vi "S2DS_EditFormula.vi"(8 "error in (no error)":errorcluster, 10 "WC info out":T2, 11 "formula in":string) -> (0 "error out":errorcluster, 1 "Parsed Formula Node (out)":T1, 3 "formula (out)":string)   [LabVIEW 2025]
uses:
  TYPE DEFS/S2DS_WC info.ctl
  TYPE DEFS/S2DS_Single WC info.ctl
  <vilib>/gmath/NI_Gmath.lvlib
panel:
  in  "Original formula":bool
  in  "Clear error":bool
  in  "OK":bool
  out "error":errorcluster
  in  "Quit sweep":bool
  out "Channel assignment":string[][](array[string])
  out "Output":dbl[](array[numeric]) format="%.2f"
  in  "Input":dbl[](array[numeric]) format="%.2f"
  in  "formula":string
  # "EDIT FORMULA..."
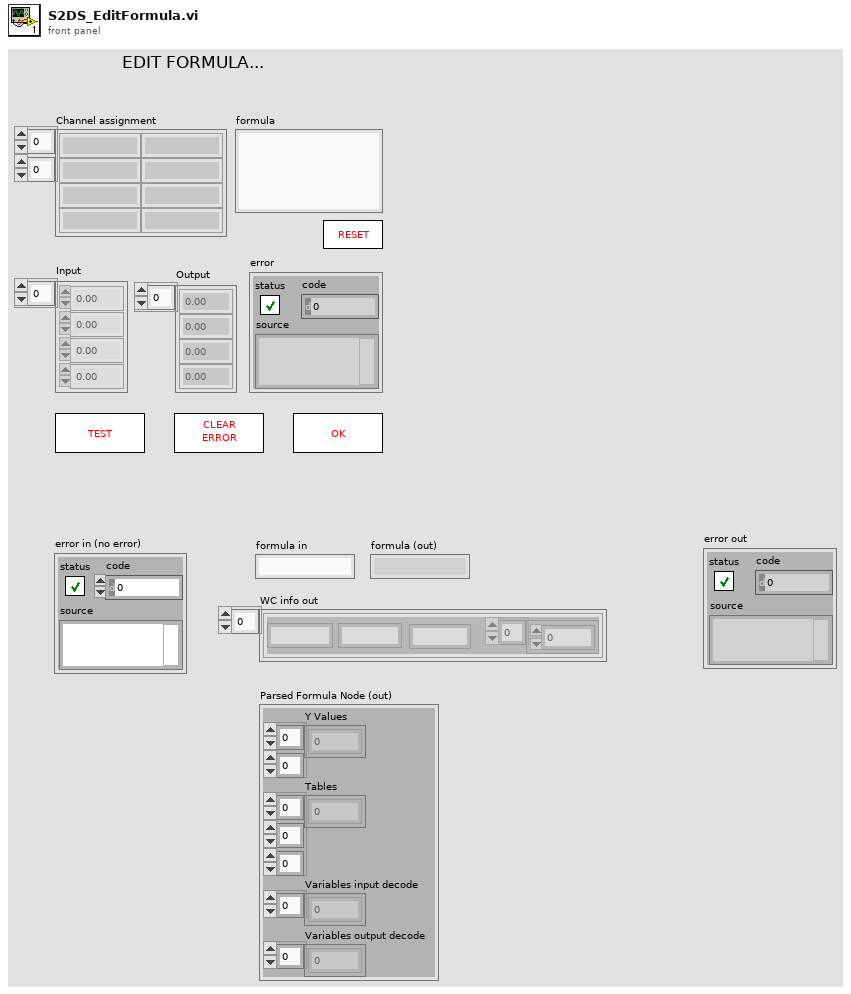
[diagram p1: front panel]
types:
  T1 = cluster{"Y Values":dbl[][], "Tables":i32[][][], "Variables input decode":i32[], "Variables output decode":i32[]}
  T2 = typedef "S2DS_WC info.ctl" = T3[]
  T3 = typedef "S2DS_Single WC info.ctl" = cluster{"Instrument identifier":string, "Write channel parameters":dbl[], "Name":string, "Unit":string}
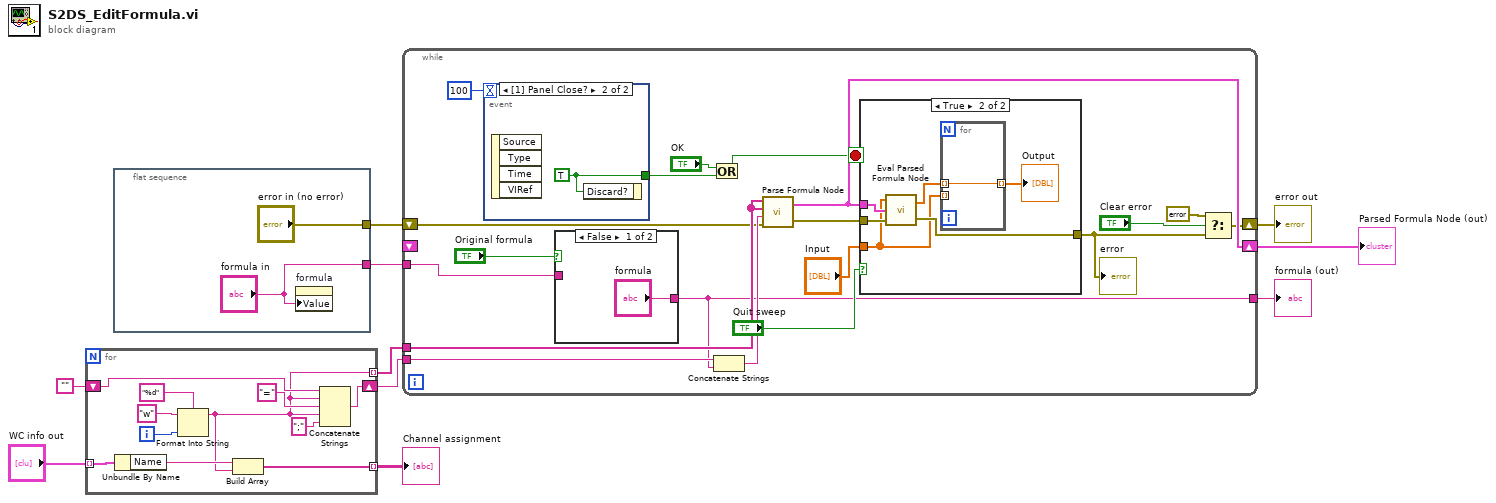
[diagram p0: block diagram]
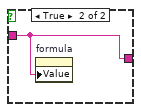
[diagram p2: hidden frame]
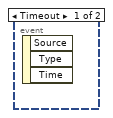
[diagram p4: hidden frame]
diagram:
  n1 = for {
    tunnel: [w12] -> w10 mode=indexing
    shift-right: [w15] -> w8
    shift-left: "" -> [w16]
    tunnel: "WC info out" -> [w14] mode=indexing
    tunnel: [w11] -> w6 mode=indexing
    i -> [w21]
    n2 = Unbundle By Name(w14) -> ("Name"=w13:string)
    n3 = Format Into String(format string="%d", initial string="w", w21) -> (resulting string=w12:string)  [unwired: 1 in, 1 out]
    n4 = Build Array(w13, w12) -> (w11:string[])
    n5 = Concatenate Strings(w16, w12, "=" ("string"), w12, ";" ("string")) -> (w15:string)
  }
  "Channel assignment" <- w6
  n6 = flat-sequence {
    tunnel: ["error in (no error)"] -> w5
    tunnel: ["formula in"] -> w1
    frame #0 {
      n7 = property on="formula" class="Str"("Value"="formula in") -> ()  [unwired: 2 in, 2 out]
    }
  }
  n8 = while {
    tunnel: w10 -> [w40]
    tunnel: w8 -> [w39]
    shift-right: [w28] -> w4
    shift-left: w5 -> [w36]
    shift-right: [w35] -> w3
    shift-left: _ -> [_]
    tunnel: [w24] -> w2
    tunnel: w1 -> [w25]
    stop <- w31 stop-if-true
    n9 = event shown="[1] Panel Close?" {
      selector: _ -> [_ _]
      dyn-events: _ -> [_ _]
      timeout: 100 -> [_ _]
      tunnel: [_ w53] -> w32
      event Timeout {
        n10 = event-data() -> ()  [unwired: 1 in, 3 out]
      }
      event Panel Close? {
        w53 = TRUE ("Discard?")
        n11 = event-data() -> ()  [unwired: 1 in, 4 out]
        n12 = event-data("Discard?"=w53) -> ()  [unwired: 1 in, 1 out]
      }
    }
    n13 = case shown="False" "Original formula" {
      tunnel: w25 -> [_ w44]
      tunnel: ["formula" w44] -> w24
      frame False {
      }
      frame True {
        n14 = property on="formula" class="Str"("Value"=w44) -> ()  [unwired: 2 in, 2 out]
      }
    }
    n15 = Or(x="OK", y=w32) -> (x .or. y?=w31:bool)
    n16 = Concatenate Strings(w39, w24) -> (w38:string)
    n17 = call <vilib>:"Parse Formula Node.vi"("error in (no error)"=w36, "formula"=w38, "Variables Output"=w40, "Variables Input"=w40) -> ("error out"=w41:errorcluster, "Parsed Formula Node"=w35:T1)
    n18 = case shown="True" "Quit sweep" {
      tunnel: w35 -> [_ w49]
      tunnel: "Input" -> [_ w48]
      tunnel: w41 -> [w45 w51]
      tunnel: [w45 w50] -> w29
      frame False {
      }
      frame True {
        n19 = call <vilib>:"Eval Parsed Formula Node.vi"("error in (no error)"=w51, "Parsed Formula Node"=w49, "Input Values"=w48) -> ("error out"=w50:errorcluster, "Output Values"=w47:dbl[])
        n20 = for {
          tunnel: w48 -> [_] mode=indexing
          tunnel: w47 -> [w52] mode=indexing
          tunnel: [w52] -> w46 mode=indexing
        }
        "Output" <- w46
      }
    }
    "error" <- w29
    n21 = Select(t=errorcluster {"status"=FALSE, "code"=0, "source"=""}, s="Clear error", f=w29) -> (s? t:f=w28:errorcluster)
  }
  "error out" <- w4
  "Parsed Formula Node (out)" <- w3
  "formula (out)" <- w2
